vi "ToData.vi"(8 "error in (no error)":errorcluster, 11 "E55555 in":refnum<class "E55555.lvclass">) -> (0 "error out":errorcluster, 2 "Data":string, 3 "E55555 out":refnum<class "E55555.lvclass">)   [LabVIEW 2022 SP3, in "Demo.lvlib" / "E55555.lvclass"]
uses:
  E55555.lvclass
  E55555.lvclass/E55555.ctl
  <vilib>/Utility/error.llb/Trim Whitespace One-Sided.vi
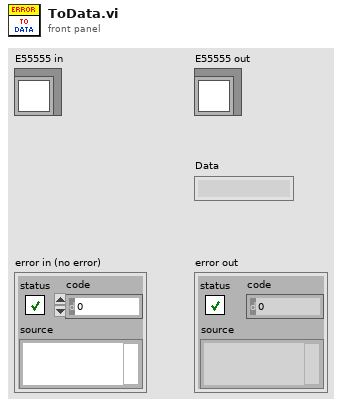
[diagram p1: front panel]
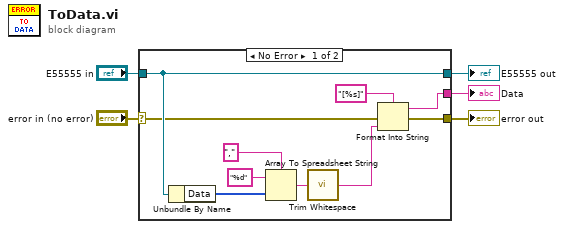
[diagram p0: block diagram]
diagram:
  n1 = case shown="No Error" "error in (no error)" {
    selector: "error in (no error)" -> [w8 w17]
    tunnel: [w7 w17] -> w5
    tunnel: [w6 _] -> w4
    tunnel: [w15 w16] -> w3
    tunnel: "E55555 in" -> [w15 w16]
    frame No Error {
      n2 = Unbundle By Name(w15) -> ("Data"=w14:i32[])
      n3 = Array To Spreadsheet String(delimiter (Tab)=",", array=w14, 3:"%d" ("format string")) -> (spreadsheet string=w11:string)
      n4 = call <vilib>:"Trim Whitespace.vi"("string"=w11) -> ("trimmed string"=w10:string)  [unwired: 1 in]
      n5 = Format Into String(format string="[%s]", error in=w8, w10) -> (resulting string=w6:string, error out=w7:errorcluster)  [unwired: 1 in]
    }
    frame Error {
    }
  }
  "error out" <- w5
  "E55555 out" <- w3
  "Data" <- w4
